vi "Delta robot kinematic.vi"(4 "re":dbl=224.0 format="%#_13g", 5 "rf":dbl=144.0 format="%#_13g", 6 "e":dbl=39.092 format="%#_13g", 7 "f":dbl=63.127 format="%#_13g", 8 "theta3":dbl, 9 "theta2":dbl, 10 "theta1":dbl) -> (0 "z0":dbl, 1 "y0":dbl format="%.5f", 2 "x0":dbl, 3 "non-existing point":bool)   [LabVIEW 2019]
panel:
  out "d":dbl
  out "d?":dbl
  out "c":dbl
  out "b":dbl
  out "a":dbl
  out "b2":dbl
  out "a2":dbl
  out "b1":dbl
  out "a1":dbl
  out "w3":dbl
  out "w2":dbl
  out "w1":dbl
  out "dnm":dbl
  out "z3":dbl
  out "x3":dbl
  out "y3":dbl
  out "z2":dbl
  out "x2":dbl
  out "y2":dbl
  out "z1":dbl
  out "y1":dbl
  out "t":dbl
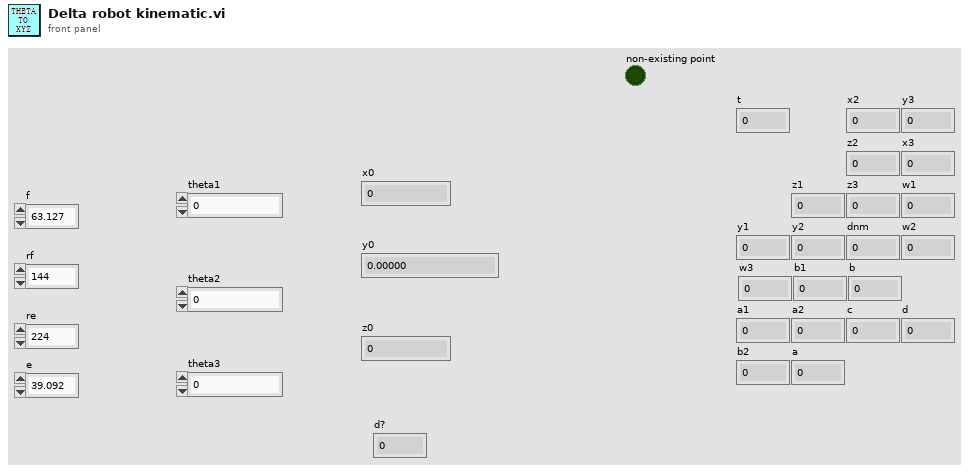
[diagram p1: front panel]
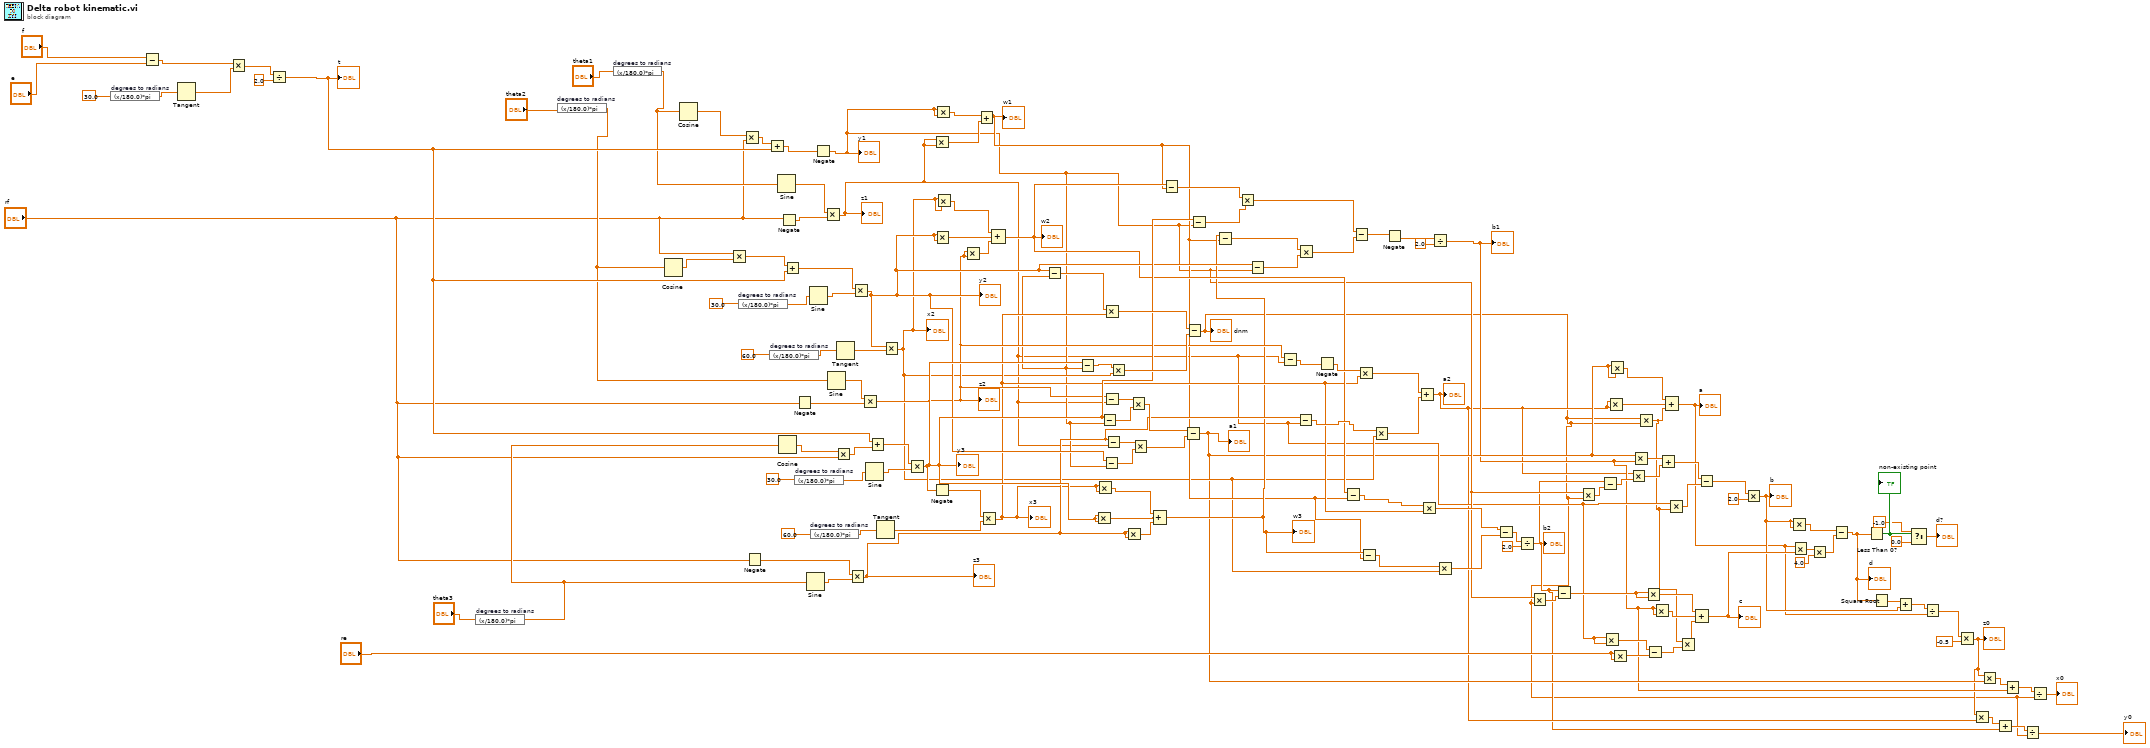
[diagram p0: block diagram]
diagram:
  n1 = expression code="(x/180.0)*pi" "degrees to radians"(30.0 ("x")) -> (w137:dbl)
  n2 = Subtract(x="f", y="e") -> (x-y=w139:dbl)
  n3 = Tangent(1:w137) -> (0:w136:dbl)
  n4 = Multiply(x=w139, y=w136) -> (x*y=w135:dbl)
  n5 = Divide(x=w135, y=2.0) -> (x/y=w115:dbl)
  "t" <- w115
  n6 = expression code="(x/180.0)*pi" "degrees to radians"("theta3") -> (w2:dbl)
  n7 = expression code="(x/180.0)*pi" "degrees to radians"("theta2") -> (w4:dbl)
  n8 = expression code="(x/180.0)*pi" "degrees to radians"("theta1") -> (w6:dbl)
  n9 = Cosine(x=w4) -> (cos(x)=w128:dbl)
  n10 = Cosine(x=w6) -> (cos(x)=w132:dbl)
  n11 = Multiply(x="rf", y=w128) -> (x*y=w127:dbl)
  n12 = expression code="(x/180.0)*pi" "degrees to radians"(30.0 ("x")) -> (w123:dbl)
  n13 = Multiply(x=w132, y="rf") -> (x*y=w133:dbl)
  n14 = Negate(x="rf") -> (-x=w105:dbl)
  n15 = Add(x=w133, y=w115) -> (x+y=w131:dbl)
  n16 = expression code="(x/180.0)*pi" "degrees to radians"(60.0 ("x")) -> (w122:dbl)
  n17 = Sine(x=w6) -> (sin(x)=w129:dbl)
  n18 = Cosine(x=w2) -> (cos(x)=w117:dbl)
  n19 = Negate(x="rf") -> (-x=w130:dbl)
  n20 = Add(x=w127, y=w115) -> (x+y=w126:dbl)
  n21 = expression code="(x/180.0)*pi" "degrees to radians"(30.0 ("x")) -> (w114:dbl)
  n22 = Negate(x="rf") -> (-x=w119:dbl)
  n23 = Sine(x=w2) -> (sin(x)=w106:dbl)
  n24 = Sine(x=w123) -> (sin(x)=w125:dbl)
  n25 = expression code="(x/180.0)*pi" "degrees to radians"(60.0 ("x")) -> (w110:dbl)
  n26 = Negate(x=w131) -> (-x=w46:dbl)
  "y1" <- w46
  n27 = Multiply(x=w129, y=w130) -> (x*y=w42:dbl)
  "z1" <- w42
  n28 = Sine(x=w4) -> (sin(x)=w118:dbl)
  n29 = Multiply(x=w117, y="rf") -> (x*y=w116:dbl)
  n30 = Tangent(1:w122) -> (0:w120:dbl)
  n31 = Multiply(x=w105, y=w106) -> (x*y=w69:dbl)
  "z3" <- w69
  n32 = Multiply(x=w126, y=w125) -> (x*y=w79:dbl)
  "y2" <- w79
  n33 = Multiply(x=w118, y=w119) -> (x*y=w75:dbl)
  "z2" <- w75
  n34 = Sine(x=w114) -> (sin(x)=w112:dbl)
  n35 = Add(x=w115, y=w116) -> (x+y=w111:dbl)
  n36 = Tangent(1:w110) -> (0:w108:dbl)
  n37 = Multiply(x=w79, y=w120) -> (x*y=w60:dbl)
  "x2" <- w60
  n38 = Multiply(x=w111, y=w112) -> (x*y=w84:dbl)
  "y3" <- w84
  n39 = Multiply(x=w42, y=w42) -> (x*y=w99:dbl)
  n40 = Negate(x=w84) -> (-x=w107:dbl)
  n41 = Multiply(x=w79, y=w79) -> (x*y=w97:dbl)
  n42 = Multiply(x=w46, y=w46) -> (x*y=w100:dbl)
  n43 = Multiply(x=w60, y=w60) -> (x*y=w98:dbl)
  n44 = Multiply(x=w75, y=w75) -> (x*y=w96:dbl)
  n45 = Add(x=w100, y=w99) -> (x+y=w61:dbl)
  "w1" <- w61
  n46 = Multiply(x=w107, y=w108) -> (x*y=w63:dbl)
  "x3" <- w63
  n47 = Compound Arithmetic op=ADD(w98, w97, w96) -> (w65:dbl)
  "w2" <- w65
  n48 = Subtract(x=w79, y=w46) -> (x-y=w104:dbl)
  n49 = Subtract(x=w84, y=w46) -> (x-y=w102:dbl)
  n50 = Multiply(x=w84, y=w84) -> (x*y=w94:dbl)
  n51 = Multiply(x=w63, y=w63) -> (x*y=w93:dbl)
  n52 = Subtract(x=w84, y=w46) -> (x-y=w91:dbl)
  n53 = Subtract(x=w79, y=w46) -> (x-y=w89:dbl)
  n54 = Multiply(x=w104, y=w63) -> (x*y=w103:dbl)
  n55 = Subtract(x=w75, y=w42) -> (x-y=w92:dbl)
  n56 = Subtract(x=w69, y=w42) -> (x-y=w88:dbl)
  n57 = Multiply(x=w102, y=w60) -> (x*y=w101:dbl)
  n58 = Multiply(x=w69, y=w69) -> (x*y=w95:dbl)
  n59 = Multiply(x=w92, y=w91) -> (x*y=w90:dbl)
  n60 = Multiply(x=w88, y=w89) -> (x*y=w87:dbl)
  n61 = Compound Arithmetic op=ADD(w93, w94, w95) -> (w62:dbl)
  "w3" <- w62
  n62 = Subtract(x=w65, y=w61) -> (x-y=w86:dbl)
  n63 = Subtract(x=w90, y=w87) -> (x-y=w17:dbl)
  "a1" <- w17
  n64 = Subtract(x=w103, y=w101) -> (x-y=w9:dbl)
  "dnm" <- w9
  n65 = Subtract(x=w84, y=w46) -> (x-y=w85:dbl)
  n66 = Subtract(x=w62, y=w61) -> (x-y=w81:dbl)
  n67 = Multiply(x=w86, y=w85) -> (x*y=w83:dbl)
  n68 = Subtract(x=w79, y=w46) -> (x-y=w82:dbl)
  n69 = Subtract(x=w75, y=w42) -> (x-y=w74:dbl)
  n70 = Subtract(x=w69, y=w42) -> (x-y=w71:dbl)
  n71 = Multiply(x=w81, y=w82) -> (x*y=w80:dbl)
  n72 = Negate(x=w74) -> (-x=w73:dbl)
  n73 = Subtract(x=w65, y=w61) -> (x-y=w64:dbl)
  n74 = Subtract(x=w83, y=w80) -> (x-y=w78:dbl)
  n75 = Multiply(x=w73, y=w63) -> (x*y=w72:dbl)
  n76 = Subtract(x=w62, y=w61) -> (x-y=w68:dbl)
  n77 = Multiply(x=w71, y=w60) -> (x*y=w70:dbl)
  n78 = Negate(x=w78) -> (-x=w77:dbl)
  n79 = Add(x=w72, y=w70) -> (x+y=w11:dbl)
  "a2" <- w11
  n80 = Multiply(x=w64, y=w63) -> (x*y=w67:dbl)
  n81 = Divide(x=w77, y=2.0) -> (x/y=w16:dbl)
  "b1" <- w16
  n82 = Multiply(x=w68, y=w60) -> (x*y=w66:dbl)
  n83 = Subtract(x=w67, y=w66) -> (x-y=w58:dbl)
  n84 = Divide(x=w58, y=2.0) -> (x/y=w10:dbl)
  "b2" <- w10
  n85 = Multiply(x=w46, y=w9) -> (x*y=w47:dbl)
  n86 = Subtract(x=w10, y=w47) -> (x-y=w45:dbl)
  n87 = Multiply(x=w46, y=w9) -> (x*y=w53:dbl)
  n88 = Subtract(x=w10, y=w53) -> (x-y=w52:dbl)
  n89 = Multiply(x=w42, y=w42) -> (x*y=w41:dbl)
  n90 = Multiply(x=w11, y=w11) -> (x*y=w57:dbl)
  n91 = Multiply(x=w17, y=w17) -> (x*y=w56:dbl)
  n92 = Multiply(x="re", y="re") -> (x*y=w40:dbl)
  n93 = Multiply(x=w11, y=w52) -> (x*y=w51:dbl)
  n94 = Multiply(x=w17, y=w16) -> (x*y=w54:dbl)
  n95 = Multiply(x=w9, y=w9) -> (x*y=w37:dbl)
  n96 = Multiply(x=w45, y=w45) -> (x*y=w44:dbl)
  n97 = Subtract(x=w41, y=w40) -> (x-y=w38:dbl)
  n98 = Multiply(x=w16, y=w16) -> (x*y=w43:dbl)
  n99 = Add(x=w54, y=w51) -> (x+y=w50:dbl)
  n100 = Compound Arithmetic op=ADD(w56, w57, w37) -> (w21:dbl)
  "a" <- w21
  n101 = Multiply(x=w42, y=w37) -> (x*y=w49:dbl)
  n102 = Multiply(x=w37, y=w38) -> (x*y=w36:dbl)
  n103 = Compound Arithmetic op=ADD(w44, w43, w36) -> (w31:dbl)
  "c" <- w31
  n104 = Subtract(x=w50, y=w49) -> (x-y=w48:dbl)
  n105 = Multiply(x=w48, y=2.0) -> (x*y=w23:dbl)
  "b" <- w23
  n106 = Multiply(x=w23, y=w23) -> (x*y=w35:dbl)
  n107 = Multiply(x=w21, y=w31) -> (x*y=w34:dbl)
  n108 = Multiply(x=w34, y=4.0) -> (x*y=w33:dbl)
  n109 = Subtract(x=w35, y=w33) -> (x-y=w25:dbl)
  "d" <- w25
  n110 = Less Than 0?(x=w25) -> (x < 0?=w30:bool)
  "non-existing point" <- w30
  n111 = Square Root(x=w25) -> (sqrt(x)=w24:dbl)
  n112 = Add(x=w24, y=w23) -> (x+y=w22:dbl)
  n113 = Select(t=-1.0, s=w30, f=0.0) -> (s? t:f=→"d?":dbl)
  n114 = Divide(x=w22, y=w21) -> (x/y=w20:dbl)
  n115 = Multiply(x=w20, y=-0.5) -> (x*y=w12:dbl)
  "z0" <- w12
  n116 = Multiply(x=w12, y=w11) -> (x*y=w14:dbl)
  n117 = Multiply(x=w12, y=w17) -> (x*y=w18:dbl)
  n118 = Add(x=w14, y=w10) -> (x+y=w13:dbl)
  n119 = Add(x=w18, y=w16) -> (x+y=w19:dbl)
  n120 = Divide(x=w13, y=w9) -> (x/y=→"y0":dbl)
  n121 = Divide(x=w19, y=w9) -> (x/y=→"x0":dbl)
